vi "ErrorPopup.vi"(8 "error in (no error)":errorcluster) -> (0 "error out":errorcluster)   [LabVIEW 2014, in "GRBLMotionCore.lvlib"]
uses:
  <instrlib>/GRBL/GRBLMotionCore.lvlib
panel:
  in  "Clear":bool
  out "Error source":string
  in  "Stop":bool
  in  "Ignore":bool
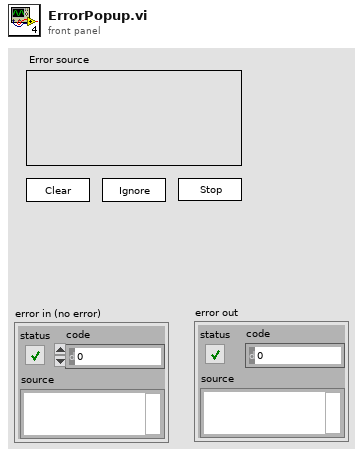
[diagram p1: front panel]
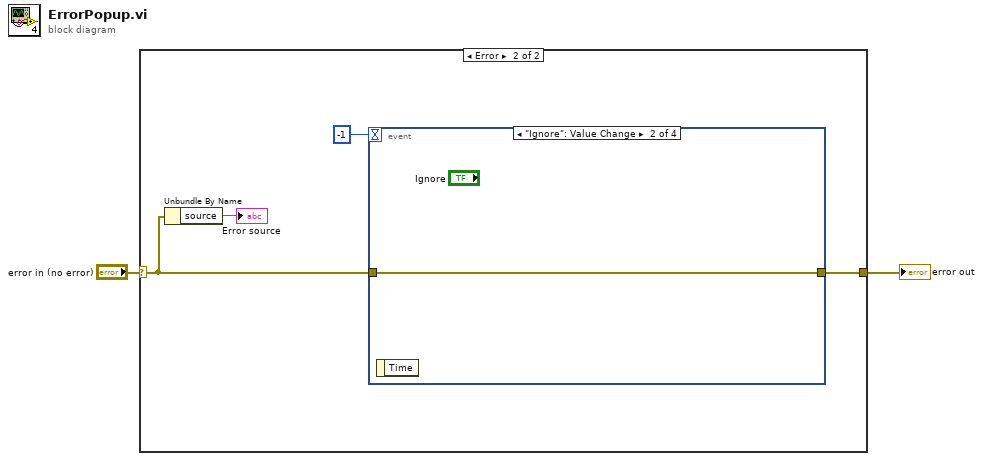
[diagram p0: block diagram]
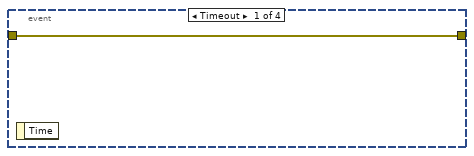
[diagram p3: hidden frame]
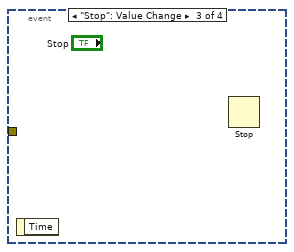
[diagram p4: hidden frame]
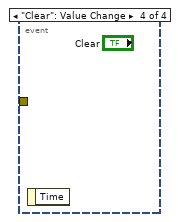
[diagram p5: hidden frame]
diagram:
  n1 = case shown="Error" "error in (no error)" {
    selector: "error in (no error)" -> [w3 w6]
    tunnel: [w3 w7] -> w1
    frame No Error {
    }
    frame Error {
      n2 = Unbundle By Name(w6) -> ("source"=→"Error source":string)
      n3 = event shown="[1] \"Ignore\": Value Change" {
        selector: _ -> [_ _ _ _]
        dyn-events: _ -> [_ _ _ _]
        timeout: -1 -> [_ _ _ _]
        tunnel: [w8 w9 _ _] -> w7
        tunnel: w6 -> [w8 w9 _ _]
        event Timeout {
          n4 = event-data() -> ()  [unwired: 1 in, 1 out]
        }
        event "Ignore": Value Change {
          n5 = event-data() -> ()  [unwired: 1 in, 1 out]
        }
        event "Stop": Value Change {
          n6 = event-data() -> ()  [unwired: 1 in, 1 out]
          n7 = Stop() -> ()  [unwired: 1 in]
        }
        event "Clear": Value Change {
          n8 = event-data() -> ()  [unwired: 1 in, 1 out]
        }
      }
    }
  }
  "error out" <- w1
